vi "spill_param_tcp_query_v2.vi"(6 "time_out":i32=100, 9 "n_try":i32=2) -> (0 "status":bool, 1 "spill_id":i32=-1, 2 "EOS":bool, 3 "BOS":bool)   [LabVIEW 2019]
panel:
  out "client_step":i32
  out "error out":errorcluster
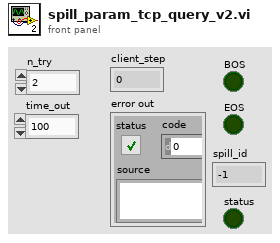
[diagram p1: front panel]
types:
  T1 = enum16{"Standard", "Buffered", "CRLF", "Immediate"}
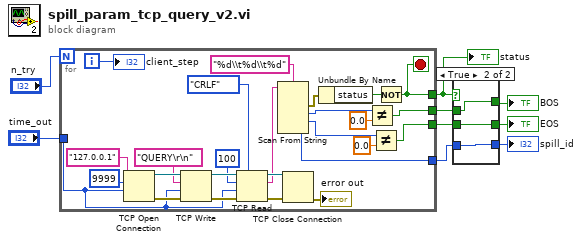
[diagram p0: block diagram]
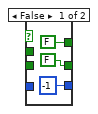
[diagram p2: hidden frame]
diagram:
  n1 = for {
    N: "n_try" -> [_]
    tunnel: "time_out" -> [w17]
    tunnel: [w18] -> w6
    tunnel: [w14] -> w4
    tunnel: [w11] -> w3
    tunnel: [w10] -> w2
    i -> [w20]
    stop <- w18 stop-if-true
    n2 = TCP Open Connection(address="127.0.0.1", remote port or service name=u16 9999, timeout ms (60000)=w17) -> (connection ID=w33:refnum<k5>, error out=w32:errorcluster)  [unwired: 2 in]
    n3 = TCP Write(connection ID=w33, data in="QUERY\r\n", error in (no error)=w32, 9:w17) -> (connection ID out=w29:refnum<k5>, error out=w30:errorcluster)  [unwired: 1 out]
    n4 = TCP Read(connection ID=w29, bytes to read=100, error in (no error)=w30, 7:T1."CRLF" ("mode (standard)"), 9:w17) -> (connection ID out=w27:refnum<k5>, data out=w25:string, error out=w28:errorcluster)
    n5 = Scan From String(format string="%d\\t%d\\t%d", input string=w25) -> (error out=w23:errorcluster, output 1=w15:i32, output 2=w12:i32, output 3=w10:i32)  [unwired: 5 in, 2 out]
    n6 = TCP Close Connection(connection ID=w27, error in (no error)=w28) -> (error out=→"error out":errorcluster)  [unwired: 1 in, 1 out]
    n7 = Unbundle By Name(w23) -> ("status"=w19:bool)
    n8 = Not Equal?(x=w15, y=0.0) -> (x != y?=w14:bool)
    n9 = Not Equal?(x=w12, y=0.0) -> (x != y?=w11:bool)
    n10 = Not(x=w19) -> (.not. x?=w18:bool)
    "client_step" <- w20
  }
  "status" <- w6
  n11 = case shown="True" w6 {
    tunnel: [-1 w41] -> w7
    tunnel: w2 -> [_ w41]
    tunnel: [FALSE w40] -> w1
    tunnel: [FALSE w39] -> w5
    tunnel: w4 -> [_ w40]
    tunnel: w3 -> [_ w39]
    frame False {
    }
    frame True {
    }
  }
  "spill_id" <- w7
  "BOS" <- w1
  "EOS" <- w5
